vi "Close_Connection.vi"(8 "error in (no error)":errorcluster, 11 "NXP in":refnum<class "NXP.lvclass">) -> (0 "error out":errorcluster, 3 "NXP out":refnum<class "NXP.lvclass">)   [LabVIEW 2019, in "NXP.lvclass"]
doc: "Close the connection with the NXP MCU"
uses:
  NXP.lvclass
  Clase Padre/Serial Device.lvclass
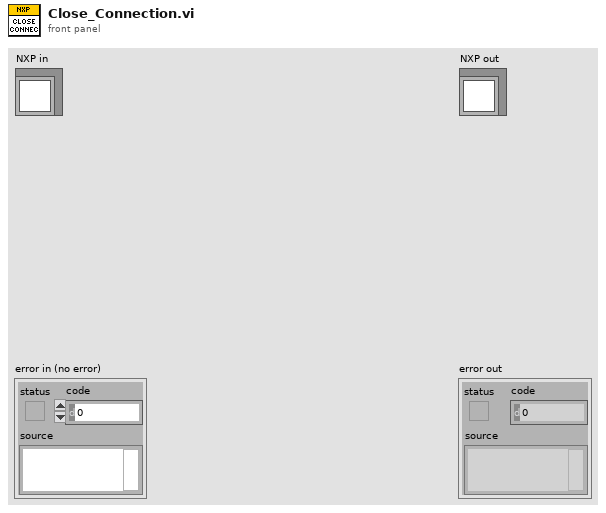
[diagram p1: front panel]
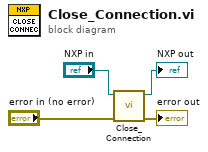
[diagram p0: block diagram]
diagram:
  n1 = call-parent "Close_Connection.vi"("error in (no error)"="error in (no error)", "Serial Device in"="NXP in") -> ("error out"=→"error out":errorcluster, "Serial Device out"=→"NXP out":refnum<class "NXP.lvclass">)  [unwired: 8 in]
